vi "Parse Results.vi"(11 "body":string) -> (3 "test results":T1)   [LabVIEW 2019]
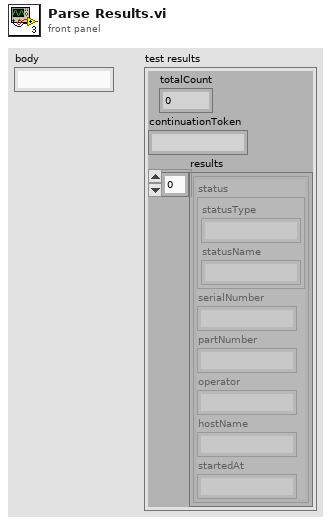
[diagram p1: front panel]
types:
  T1 = cluster{"totalCount":i32, "continuationToken":string, "results":cluster{"status":cluster{"statusType":string, "statusName":string}, "serialNumber":string, "partNumber":string, "operator":string, "hostName":string, "startedAt":string}[]}
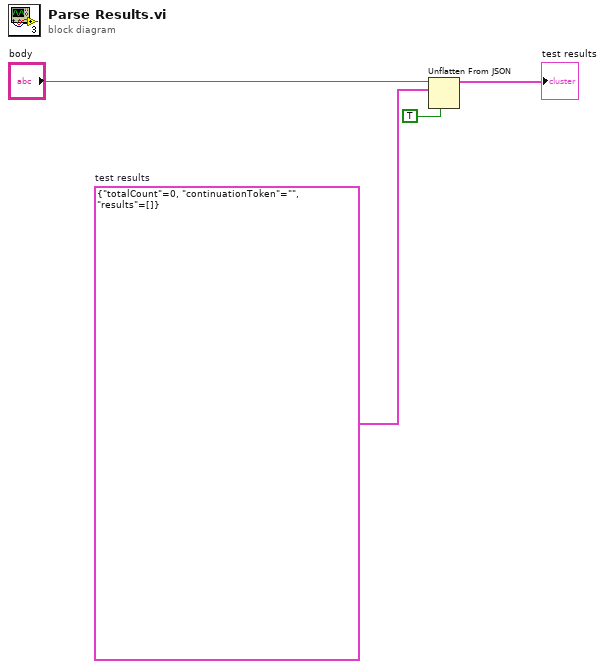
[diagram p0: block diagram]
diagram:
  w1 = T1 {"totalCount"=0, "continuationToken"="", "results"=[]}  # test results
  n1 = Unflatten From JSON(JSON string="body", type and defaults=w1, default null elements? (F)=TRUE) -> (value=→"test results":T1)  [unwired: 4 in, 1 out]
